vi "Set Connection.vi"(8 "error in (no error)":errorcluster, 11 "connection":T1) -> (0 "error out":errorcluster)   [LabVIEW 2021, in "AudioGenManageConnection.lvlib"]
uses:
  <vilib>/NI/STM/TCP/TCP Connection Info.ctl
  <vilib>/NI/STM/SubVIs/MetaDataElement.ctl
  <vilib>/addons/PointValueMap/subVIs/Point_Write_variant.vi
  AudioGenManageConnection.lvlib
  <vilib>/addons/PointValueMap/PointValueMap.lvlib
  <vilib>/NI/STM/NI STM.lvlib
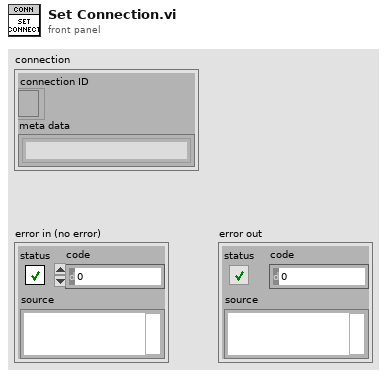
[diagram p1: front panel]
types:
  T1 = typedef "NI STM.lvlib/TCP Connection Info.ctl" = cluster{"connection ID":refnum<k5>, "meta data":T2[]}
  T2 = typedef "NI STM.lvlib/MetaDataElement.ctl" = string
  T3 = typedef "PointValueMap.lvlib/PointMap.ctl" = refnum<data-value>
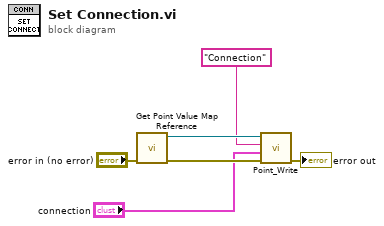
[diagram p0: block diagram]
diagram:
  n1 = call "Get Point Value Map Reference.vi"("error in (no error)"="error in (no error)") -> ("error out"=w4:errorcluster, "Map Out"=w5:T3)  [unwired: 9 in]
  n2 = call-poly <vilib>:"Point_Write.vi"("Error In"=w4, "Value"="connection", "Tag"="Connection", "Map"=w5) -> ("Error Out"=→"error out":errorcluster)  [unwired: 6 in, 1 out]
